vi "19.1-MovingAverageH[k]-Rect.vi"() -> ()   [LabVIEW 2020]
doc: "Uses the Median Filter VI to analyze pulses in the presence of noise. The example generates a pulse contaminated with Gaussian noise and applies a median filter. For comparison purposes, the VI computes the pulse parameters of the filtered pulse."
uses:
  <vilib>/Analysis/2dsp.llb/1D Convolution (DBL).vi
  <vilib>/Analysis/2dsp.llb/Real FFT.vi
  <vilib>/Analysis/NI_AALPro.lvlib
panel:
  out "H[k]":dbl[][](graph)
  out "h[n]":dbl[](graph) caption="h[i]"
  # "1"
  # "2"
  # "4"
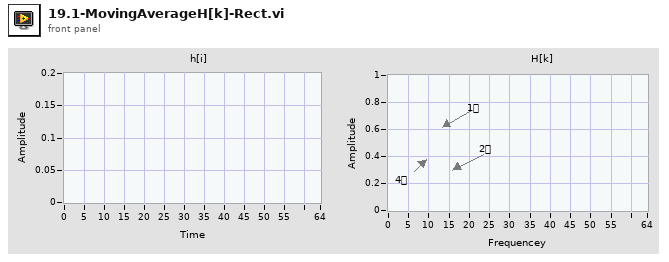
[diagram p1: front panel]
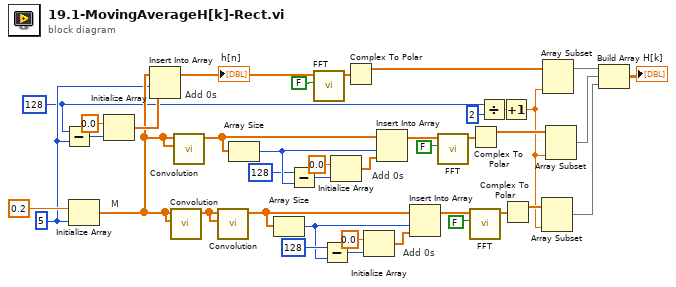
[diagram p0: block diagram]
diagram:
  w12 = 5 ("dimension size")
  w9 = 128 ("dimension size")
  # "M"
  # "Add 0s"
  # "Add 0s"
  # "Add 0s"
  n1 = Subtract(x=w9, y=w12) -> (x-y=w31:i32)
  n2 = Initialize Array(0.2 ("element"), w12) -> (w13:dbl[])
  n3 = Initialize Array(0.0 ("element"), w31) -> (w36:dbl[])
  n4 = Insert Into Array(array=w13, index=w12, new element=w36) -> (w11:dbl[])
  "h[n]" <- w11
  n5 = call-poly <vilib>:"Convolution.vi"("Y"=w13, "X"=w13) -> ("X * Y"=w33:dbl[])  [unwired: 8 in, 1 out]
  n6 = call-poly <vilib>:"Convolution.vi"("Y"=w13, "X"=w13) -> ("X * Y"=w18:dbl[])  [unwired: 8 in, 1 out]
  n7 = call-poly <vilib>:"Convolution.vi"("Y"=w33, "X"=w33) -> ("X * Y"=w32:dbl[])  [unwired: 8 in, 1 out]
  n8 = Array Size(array=w18) -> (size(s)=w22:i32)
  n9 = Array Size(array=w32) -> (size(s)=w28:i32)
  n10 = Subtract(x=128 ("dimension size"), y=w22) -> (x-y=w21:i32)
  n11 = call-poly <vilib>:"FFT.vi"("shift?"=FALSE, "X"=w11) -> ("FFT {X}"=w38:cdb[])  [unwired: 8 in, 1 out]
  n12 = Subtract(x=128 ("dimension size"), y=w28) -> (x-y=w29:i32)
  n13 = Initialize Array(0.0 ("element"), w21) -> (w24:dbl[])
  n14 = Complex To Polar(r * e^(i*theta)=w38) -> (r=w10:dbl[])  [unwired: 1 out]
  n15 = Initialize Array(0.0 ("element"), w29) -> (w26:dbl[])
  n16 = Insert Into Array(array=w18, index=w22, new element=w24) -> (w15:dbl[])
  n17 = Insert Into Array(array=w32, index=w28, new element=w26) -> (w25:dbl[])
  n18 = call-poly <vilib>:"FFT.vi"("shift?"=FALSE, "X"=w15) -> ("FFT {X}"=w17:cdb[])  [unwired: 8 in, 1 out]
  n19 = call-poly <vilib>:"FFT.vi"("shift?"=FALSE, "X"=w25) -> ("FFT {X}"=w35:cdb[])  [unwired: 8 in, 1 out]
  n20 = Complex To Polar(r * e^(i*theta)=w17) -> (r=w5:dbl[])  [unwired: 1 out]
  n21 = Divide(x=w9, y=2) -> (x/y=w6:dbl)
  n22 = Increment(x=w6) -> (x+1=w2:dbl)
  n23 = Complex To Polar(r * e^(i*theta)=w35) -> (r=w3:dbl[])  [unwired: 1 out]
  n24 = Array Subset(array=w3, length=w2) -> (w1:dbl[])  [unwired: 1 in]
  n25 = Array Subset(array=w10, length=w2) -> (w7:dbl[])  [unwired: 1 in]
  n26 = Array Subset(array=w5, length=w2) -> (w4:dbl[])  [unwired: 1 in]
  n27 = Build Array(w7, w4, w1) -> (→"H[k]":dbl[][])
